vi "main.vi"() -> ()   [LabVIEW 2021]
uses:
  Expression.ctl
  ExpressionType.ctl
  Environment.ctl
panel:
  out "Environment out":T1
  in  "ShowType?":bool=TRUE
  out "Expression in":T2
  out "expression out":string
  out "Expression out":T2
  out "expression in":string
  in  "input string":string="progn\n  (define pi 3.14)\n  (define r 4)\n  (define h 12)\n  (* pi r r h)"
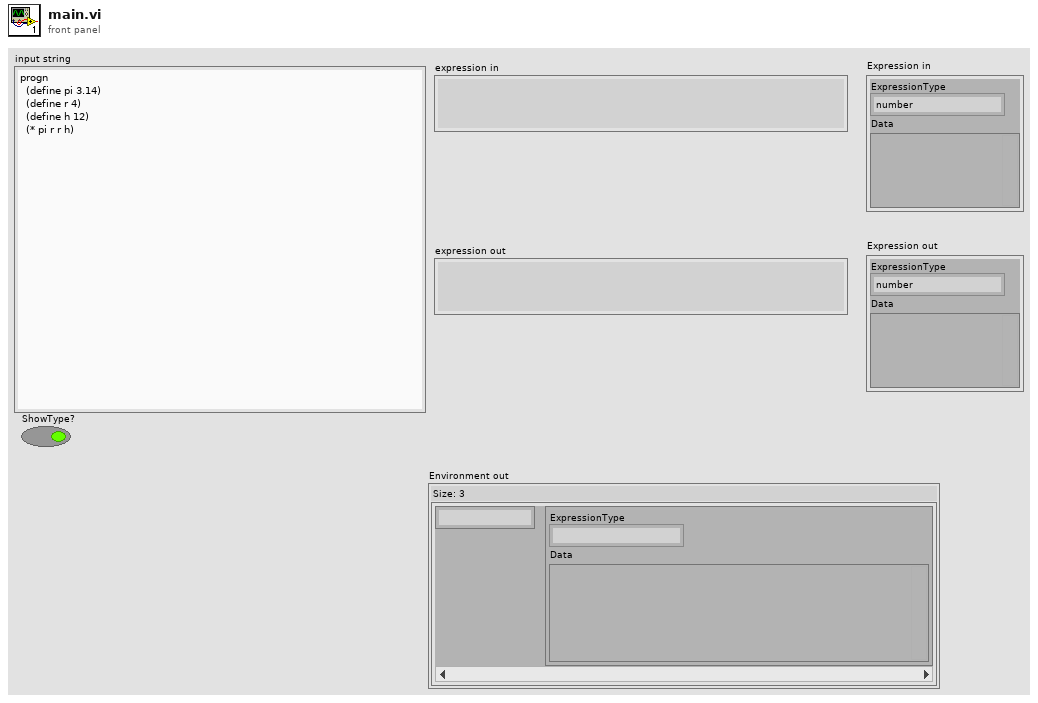
[diagram p1: front panel]
types:
  T1 = typedef "Environment.ctl" = map{string, T2}
  T2 = typedef "Expression.ctl" = cluster{"ExpressionType":T3, "Data":variant}
  T3 = typedef "ExpressionType.ctl" = enum16{"number", "string", "symbol", "primitive", "list", "closure", "nil", "error"}
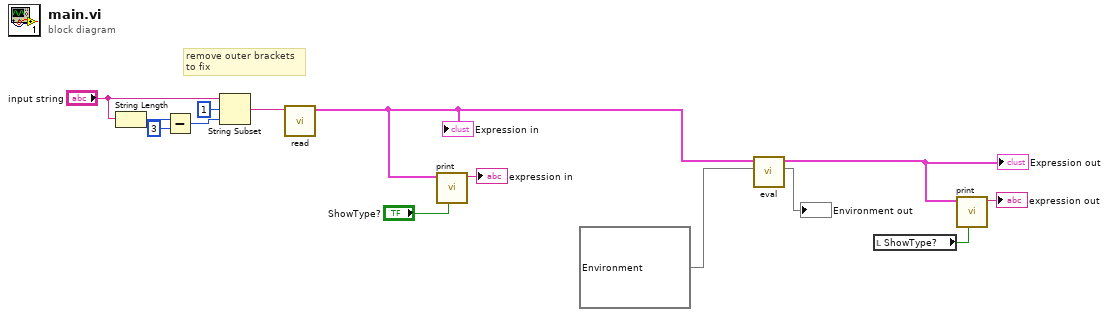
[diagram p0: block diagram]
diagram:
  # "remove outer brackets\nto fix"
  n1 = String Length(string="input string") -> (length=w3:i32)
  n2 = Subtract(x=w3, y=3) -> (x-y=w2:i32)
  n3 = String Subset(string="input string", offset (0)=1, length (rest)=w2) -> (substring=w6:string)
  n4 = call "read.vi"("input string"=w6) -> ("Expression out"=w10:T2)  [unwired: 10 in]
  "Expression in" <- w10
  n5 = call "print.vi"("ShowType?"="ShowType?", "Expression"=w10) -> ("String"=→"expression in":string)  [unwired: 8 in, 1 out]
  n6 = call "eval.vi"("Environment in"=T1 {}, "Expression in"=w10) -> ("Environment out"=→"Environment out":T1, "Expression out"=w11:T2)  [unwired: 6 in]
  "Expression out" <- w11
  n7 = local read "ShowType?"() -> (w9:bool)
  n8 = call "print.vi"("ShowType?"=w9, "Expression"=w11) -> ("String"=→"expression out":string)  [unwired: 8 in, 1 out]
